vi "Stop Connection Handler.vi"(8 "error in (no error)":errorcluster, 11 "TCPConnectionHandler in":refnum<class "TCPConnectionHandler.lvclass">) -> (0 "error out":errorcluster, 3 "TCPConnectionHandler out":refnum<class "TCPConnectionHandler.lvclass">)   [LabVIEW 2013, in "MQTT_TCP.lvlib" / "TCPConnectionHandler.lvclass"]
uses:
  TCPConnectionHandler.lvclass
  TCPConnectionHandler.lvclass/TCPConnectionHandler.ctl
panel:
  out "timed out?":bool
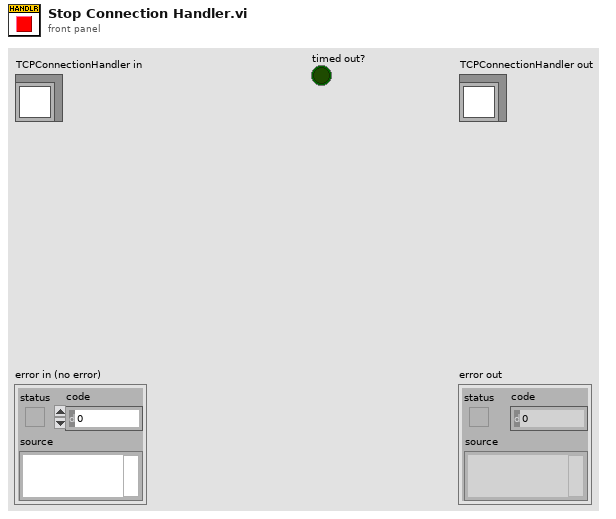
[diagram p1: front panel]
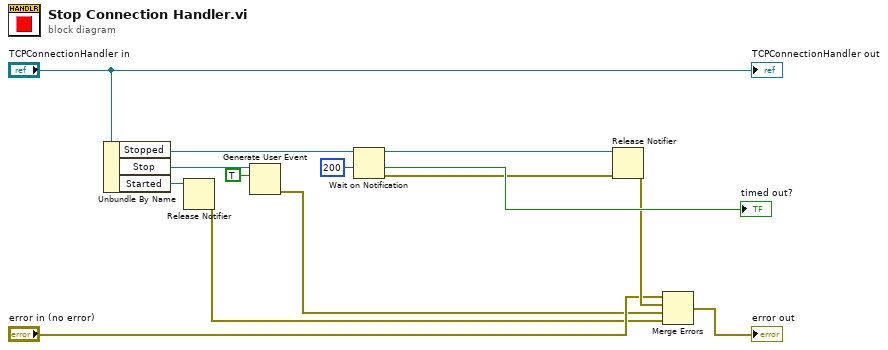
[diagram p0: block diagram]
diagram:
  n1 = Unbundle By Name("TCPConnectionHandler in") -> ("Stopped"=w10:refnum<notifier>, "Stop"=w12:refnum<user-event>, "Started"=w2:refnum<notifier>)
  n2 = Release Notifier(notifier=w2) -> (error out=w1:errorcluster)  [unwired: 2 in, 2 out]
  n3 = Generate User Event(user event=w12, event data cluster=TRUE ("event data")) -> (error out=w3:errorcluster)  [unwired: 2 in, 1 out]
  n4 = Wait on Notification(notifier=w10, timeout in ms (-1)=200) -> (notifier out=w7:refnum<notifier>, timed out?=→"timed out?":bool, error out=w8:errorcluster)  [unwired: 2 in, 1 out]
  n5 = Release Notifier(notifier=w7, error in (no error)=w8) -> (error out=w6:errorcluster)  [unwired: 1 in, 2 out]
  n6 = Merge Errors("error in (no error)", w6, w3, w1) -> (→"error out":errorcluster)
  "TCPConnectionHandler out" <- "TCPConnectionHandler in"
